vi "step1_FindStartPiece.vi"(8 "error in (no error)":errorcluster, 9 "start colour":u32(colorbox), 11 "cube in":T1) -> (0 "error out":errorcluster, 3 "cube out":T1)   [LabVIEW 2011]
doc: "Rotate cube as necessary so that the top middle piece matches the desired start colour.\n\nNo transformations are done in this VI, the operations are loaded on the the operation queue bus."
uses:
  Typedef/cube.ctl
  Typedef/face.ctl
  Typedef/operation.ctl
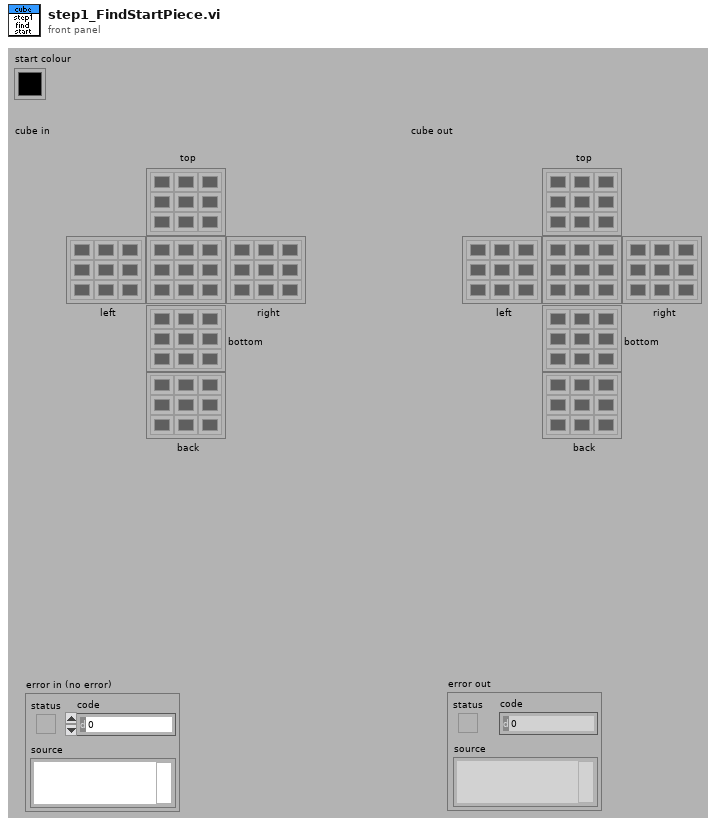
[diagram p1: front panel]
types:
  T1 = typedef "cube.ctl" = cluster{"top":T2, "left":T2, "right":T2, "bottom":T2, "back":T2, "front":T2}
  T2 = typedef "face.ctl" = u32[][]
  T3 = typedef "operation.ctl" = enum16{"nop", "T+", "T-", "F+", "F-", "L+", "L-", "R+", "R-", "B+", "B-", "<--", "-->", "^", "V"}
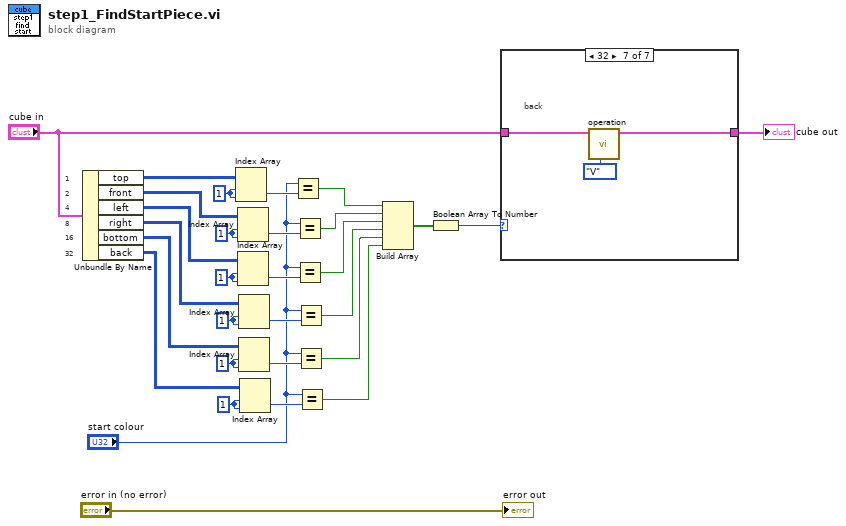
[diagram p0: block diagram]
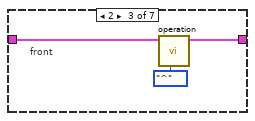
[diagram p4: hidden frame]
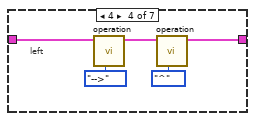
[diagram p5: hidden frame]
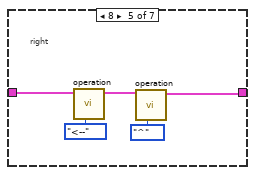
[diagram p6: hidden frame]
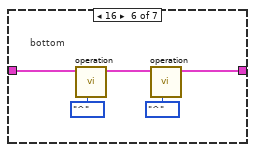
[diagram p7: hidden frame]
diagram:
  w14 = 1 ("index (row)")
  w18 = 1 ("index (row)")
  w20 = 1 ("index (row)")
  w24 = 1 ("index (row)")
  w26 = 1 ("index (row)")
  w29 = 1 ("index (row)")
  # "32"
  # "16"
  # "8"
  # "4"
  # "2"
  # "1"
  n1 = Unbundle By Name("cube in") -> ("top"=w30:T2, "front"=w25:T2, "left"=w22:T2, "right"=w19:T2, "bottom"=w16:T2, "back"=w13:T2)
  n2 = Index Array(array=w30, index (row)=w29, index (col)=w29) -> (element=w28:u32)
  n3 = Index Array(array=w25, index (row)=w26, index (col)=w26) -> (element=w27:u32)
  n4 = Index Array(array=w22, index (row)=w24, index (col)=w24) -> (element=w23:u32)
  n5 = Index Array(array=w19, index (row)=w20, index (col)=w20) -> (element=w21:u32)
  n6 = Index Array(array=w16, index (row)=w18, index (col)=w18) -> (element=w17:u32)
  n7 = Index Array(array=w13, index (row)=w14, index (col)=w14) -> (element=w15:u32)
  n8 = Equal?(x="start colour", y=w28) -> (x = y?=w11:bool)
  n9 = Equal?(x="start colour", y=w27) -> (x = y?=w10:bool)
  n10 = Equal?(x="start colour", y=w23) -> (x = y?=w9:bool)
  n11 = Equal?(x="start colour", y=w21) -> (x = y?=w8:bool)
  n12 = Equal?(x="start colour", y=w17) -> (x = y?=w7:bool)
  n13 = Equal?(x="start colour", y=w15) -> (x = y?=w6:bool)
  n14 = Build Array(w11, w10, w9, w8, w7, w6) -> (w5:bool[])
  n15 = Boolean Array To Number(Boolean array=w5) -> (number=w4:u32)
  n16 = case shown="32" w4 {
    tunnel: "cube in" -> [w31 w32 w34 w38 w43 w48 w52]
    tunnel: [w31 w32 w33 w36 w41 w46 w51] -> w1
    frame 0, Default {
      # "error!!!!"
    }
    frame 1 {
      # "top"
    }
    frame 2 {
      # "front"
      n17 = call "operation.vi"("operation"=operation."^", "cube in"=w34) -> ("cube out"=w33:T1)  [unwired: 8 in, 1 out]
    }
    frame 4 {
      # "left"
      n18 = call "operation.vi"("operation"=operation."-->", "cube in"=w38) -> ("cube out"=w37:T1)  [unwired: 8 in, 1 out]
      n19 = call "operation.vi"("operation"=operation."^", "cube in"=w37) -> ("cube out"=w36:T1)  [unwired: 8 in, 1 out]
    }
    frame 8 {
      # "right"
      n20 = call "operation.vi"("operation"=operation."<--", "cube in"=w43) -> ("cube out"=w42:T1)  [unwired: 8 in, 1 out]
      n21 = call "operation.vi"("operation"=operation."^", "cube in"=w42) -> ("cube out"=w41:T1)  [unwired: 8 in, 1 out]
    }
    frame 16 {
      # "bottom"
      n22 = call "operation.vi"("operation"=operation."^", "cube in"=w48) -> ("cube out"=w47:T1)  [unwired: 8 in, 1 out]
      n23 = call "operation.vi"("operation"=operation."^", "cube in"=w47) -> ("cube out"=w46:T1)  [unwired: 8 in, 1 out]
    }
    frame 32 {
      # "back"
      n24 = call "operation.vi"("operation"=operation."V", "cube in"=w52) -> ("cube out"=w51:T1)  [unwired: 8 in, 1 out]
    }
  }
  "cube out" <- w1
  "error out" <- "error in (no error)"
